vi "ClearMessagesControls.vi"(8 "error in (no error)":errorcluster, 11 "TCP_Client in":refnum<class "TCP_Client.lvclass">) -> (0 "error out":errorcluster, 3 "TCP_Client out":refnum<class "TCP_Client.lvclass">)   [LabVIEW 2023, in "TCP_Client.lvlib" / "TCP_Client.lvclass"]
uses:
  TCP_Client.lvclass
  TCP_Client.lvclass/TCP_Client.ctl
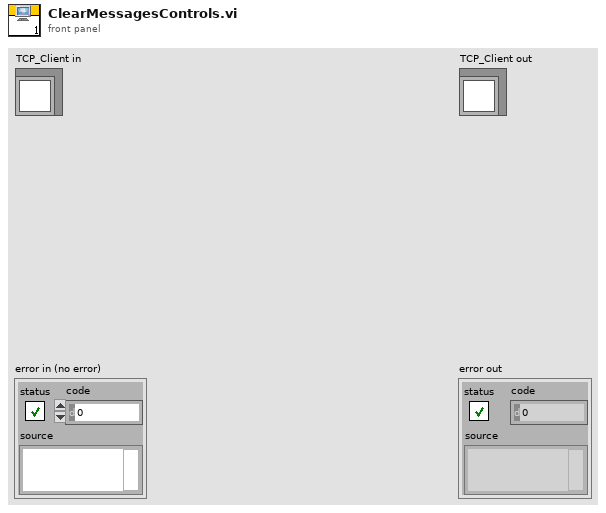
[diagram p1: front panel]
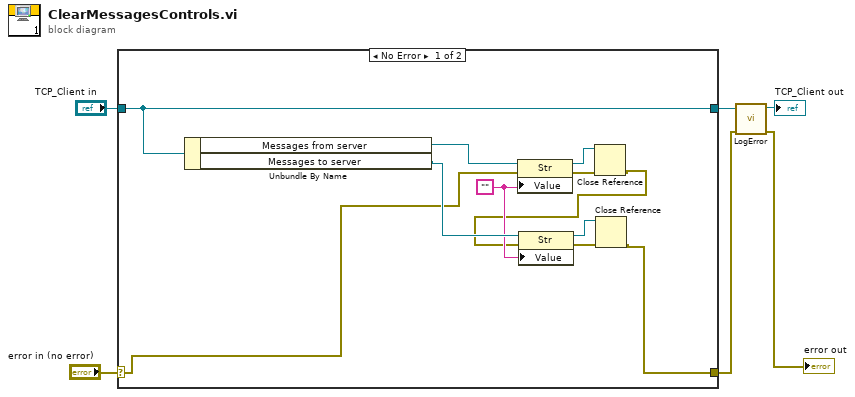
[diagram p0: block diagram]
diagram:
  n1 = case shown="No Error" "error in (no error)" {
    selector: "error in (no error)" -> [w9 w19]
    tunnel: [w7 w19] -> w2
    tunnel: [w17 w18] -> w4
    tunnel: "TCP_Client in" -> [w17 w18]
    frame No Error {
      w10 = ""
      n2 = Unbundle By Name(w17) -> ("Messages from server"=w12:refnum<vi>, "Messages to server"=w11:refnum<vi>)
      n3 = property class="Str"(reference=w12, error in=w9, "Value"=w10) -> (reference out=w15:refnum<vi>, error out=w16:errorcluster)
      n4 = Close Reference(reference=w15, error in (no error)=w16) -> (error out=w8:errorcluster)
      n5 = property class="Str"(reference=w11, error in=w8, "Value"=w10) -> (reference out=w14:refnum<vi>, error out=w13:errorcluster)
      n6 = Close Reference(reference=w14, error in (no error)=w13) -> (error out=w7:errorcluster)
    }
    frame Error {
    }
  }
  n7 = call "LogError.vi"("error in (no error)"=w2, "TCP_Client in"=w4) -> ("error out"=→"error out":errorcluster, "TCP_Client out"=→"TCP_Client out":refnum<class "TCP_Client.lvclass">)  [unwired: 8 in]
